vi "Test Example Variant Info.vi"() -> ()   [LabVIEW 2014]
panel:
  out "ClassNames":string[](array[string])
  out "objects count":i32=28
  in  "Error In":errorcluster
  in  "vi path":path=path "C:/Users/ljagos/Documents/LabVIEW/LabVIEW-Universal-Transcriptor/Test/Examples For Parsing/Example Variant Info.vi"
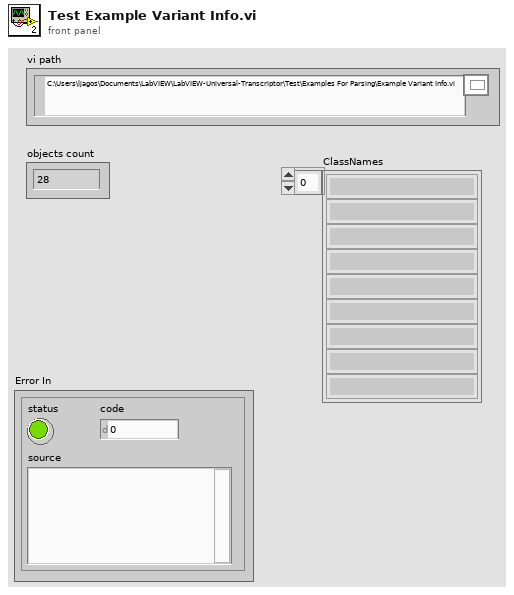
[diagram p1: front panel]
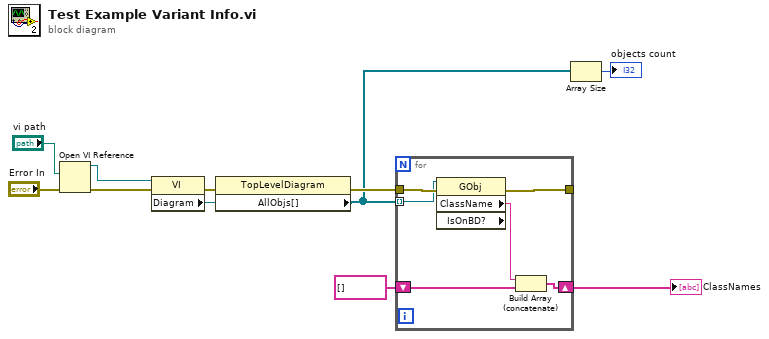
[diagram p0: block diagram]
diagram:
  n1 = Open VI Reference(vi path="vi path", error in (no error)="Error In") -> (vi reference=w3:refnum<vi>, error out=w6:errorcluster)  [unwired: 4 in]
  n2 = property class="VI"(reference=w3, error in=w6) -> (error out=w9:errorcluster, "Diagram"=w10:refnum<vi>)  [unwired: 1 out]
  n3 = property class="TopLevelDiagram"(reference=w10, error in=w9) -> (error out=w7:errorcluster, "AllObjs[]"=w4:refnum<vi>[])  [unwired: 1 out]
  n4 = for {
    tunnel: w7 -> [w17]
    tunnel: w4 -> [w16] mode=indexing
    shift-right: [w13] -> w2
    shift-left: string[] [] -> [w14]
    tunnel: [w12] -> _
    n5 = property class="GObj" props=["ClassName", "IsOnBD?"](reference=w16, error in=w17) -> (error out=w12:errorcluster, "ClassName"=w15:string)  [unwired: 2 out]
    n6 = Build Array (concatenate)(w15, w14) -> (w13:string[])
  }
  "ClassNames" <- w2
  n7 = Array Size(array=w4) -> (size(s)=→"objects count":i32)
